vi "RT_init_shared_and_network_variables.vi"(8 "error in (no error)":errorcluster) -> (0 "error out":errorcluster)   [LabVIEW 2020]
uses:
  RT_CPU_load.ctl
  RT_FIFO_Health.ctl
  RT_only_FIFO_Health.ctl
  PC_DIO_Cluster.ctl
panel:
  out "current time":timestamp
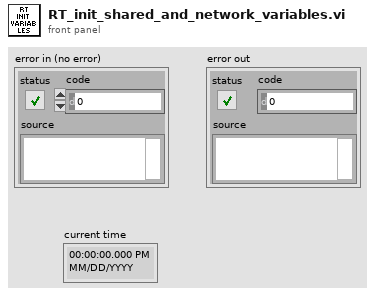
[diagram p1: front panel]
types:
  T1 = typedef "PC_DIO_Cluster.ctl" = cluster{"DIO1":bool, "DIO0":bool, "DIO2":bool, "DIO3":bool}
  T2 = typedef "RT_only_FIFO_Health.ctl" = cluster{"Elements in RT FIFO":i32, "Network Stream Full":bool, "RT FIFO Full":bool, "FPGA AI Underflow":bool, "FPGA FIFO Full":bool, "FPGA Loop Timing Off":bool, "timestamp":timestamp}
  T3 = typedef "RT_FIFO_Health.ctl" = cluster{dbl, dbl, dbl, "TotalPhysMem":dbl, "FreePhysMem":dbl, "TotalVirtMem":dbl, "FreeVirtMem":dbl, "TotalDisk":dbl, "FreeDisk":dbl}
  T4 = typedef "RT_CPU_load.ctl" = cluster{"Total (%)":dbl, "Time Critical (%)":dbl, "Timed Structures (%)":dbl, "High (%)":dbl, "Above Normal (%)":dbl, "Normal (%)":dbl, "Background (%)":dbl, "Idle (%)":dbl, "ISR (%)":dbl, "ISR (%) 2":dbl, "Idle (%) 2":dbl, "Background (%) 2":dbl, "Normal (%) 2":dbl, "Above Normal (%) 2":dbl, "High (%) 2":dbl, "Timed Structures (%) 2":dbl, "Time Critical (%) 2":dbl, "Total (%) 2":dbl}
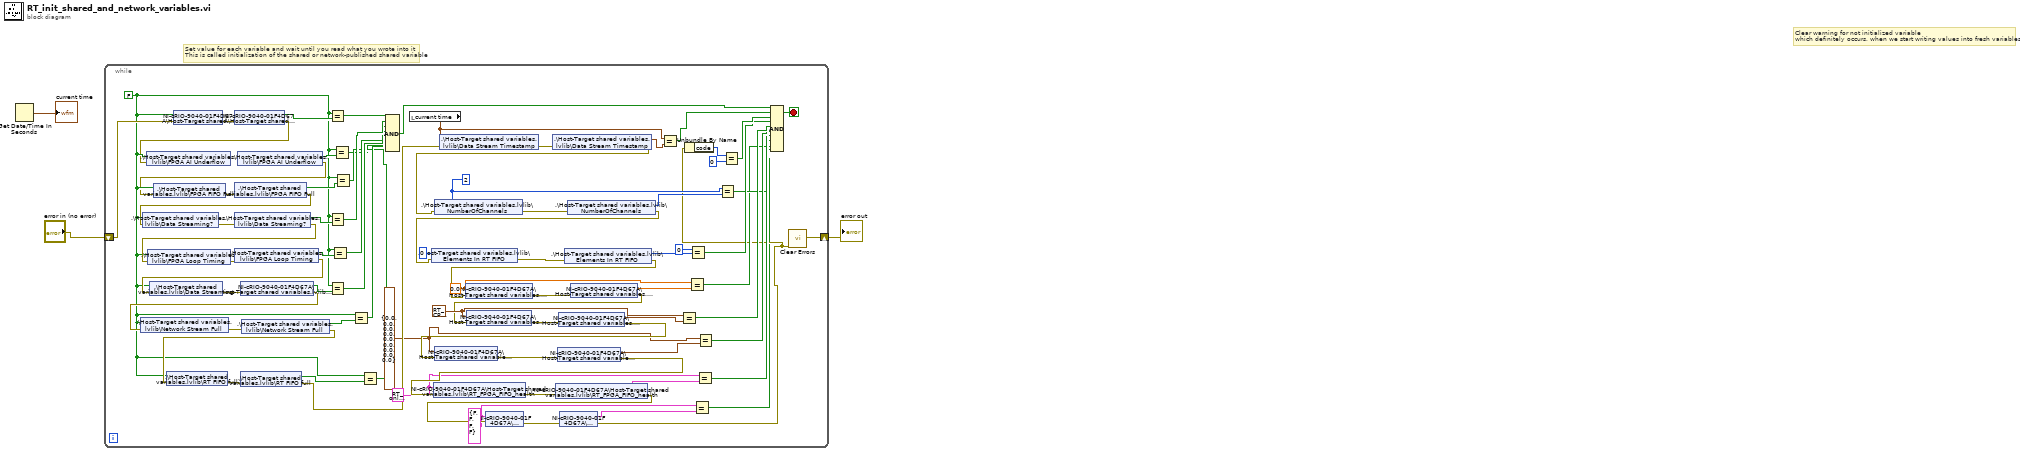
[diagram p0: block diagram]
diagram:
  # "Set value for each variable and wait until you read what you wrote into it\nThis is called initialization of the shared or network-published shared variable"
  # "Clear warning for not initialized variable\nwhich definitely occurs, when we start writing values into fresh variables"
  n1 = Get Date/Time In Seconds() -> (seconds since 1Jan1904=→"current time":timestamp)
  n2 = while {
    shift-right: [w72] -> w2
    shift-left: "error in (no error)" -> [w71]
    stop <- w65 stop-if-true
    w5 = T1 {"DIO1"=FALSE, "DIO0"=FALSE, "DIO2"=FALSE, "DIO3"=FALSE} ("DIO")
    w11 = 0.0 ("Binning Time")
    w31 = u8 2 ("NumberOfChannels")
    w37 = T2 {"Elements in RT FIFO"=0, "Network Stream Full"=FALSE, "RT FIFO Full"=FALSE, "FPGA AI Underflow"=FALSE, "FPGA FIFO Full"=FALSE, "FPGA Loop Timing Off"=FALSE, "timestamp"=timestamp(0 s since 1904-01-01)} ("RT_FIFO_health")
    w43 = T3 {0.0, 0.0, 0.0, "TotalPhysMem"=0.0, "FreePhysMem"=0.0, "TotalVirtMem"=0.0, "FreeVirtMem"=0.0, "TotalDisk"=0.0, "FreeDisk"=0.0} ("RT_FPGA_Memory_and_FIFOs")
    w46 = T4 {"Total (%)"=0.0, "Time Critical (%)"=0.0, "Timed Structures (%)"=0.0, "High (%)"=0.0, "Above Normal (%)"=0.0, "Normal (%)"=0.0, "Background (%)"=0.0, "Idle (%)"=0.0, "ISR (%)"=0.0, "ISR (%) 2"=0.0, "Idle (%) 2"=0.0, "Background (%) 2"=0.0, "Normal (%) 2"=0.0, "Above Normal (%) 2"=0.0, "High (%) 2"=0.0, "Timed Structures (%) 2"=0.0, "Time Critical (%) 2"=0.0, "Total (%) 2"=0.0} ("RT CPU Load")
    w21 = FALSE
    n3 = shared-variable "NI-cRIO-9040-01F4D67A\\Host-Target shared variables.lvlib\\Stop RT"(w21, error in=w71) -> (error out=w82:errorcluster)
    n4 = shared-variable "NI-cRIO-9040-01F4D67A\\Host-Target shared variables.lvlib\\Stop RT"(error in=w82) -> (w81:bool, error out=w19:errorcluster)
    n5 = shared-variable ".\\Host-Target shared variables.lvlib\\FPGA AI Underflow"(w21, error in=w19) -> ()  [unwired: 1 out]
    n6 = shared-variable ".\\Host-Target shared variables.lvlib\\FPGA AI Underflow"() -> (w23:bool, error out=w18:errorcluster)  [unwired: 1 in]
    n7 = shared-variable ".\\Host-Target shared variables.lvlib\\FPGA FIFO Full"(w21, error in=w18) -> (error out=w24:errorcluster)
    n8 = shared-variable ".\\Host-Target shared variables.lvlib\\FPGA FIFO Full"(error in=w24) -> (w22:bool, error out=w20:errorcluster)
    n9 = shared-variable ".\\Host-Target shared variables.lvlib\\Data Streaming?"(w21, error in=w20) -> (error out=w80:errorcluster)
    n10 = shared-variable ".\\Host-Target shared variables.lvlib\\Data Streaming?"(error in=w80) -> (w79:bool, error out=w28:errorcluster)
    n11 = shared-variable ".\\Host-Target shared variables.lvlib\\FPGA Loop Timing"(w21, error in=w28) -> (error out=w29:errorcluster)
    n12 = shared-variable ".\\Host-Target shared variables.lvlib\\FPGA Loop Timing"(error in=w29) -> (w26:bool, error out=w27:errorcluster)
    n13 = shared-variable ".\\Host-Target shared variables.lvlib\\Data Streaming"(w21, error in=w27) -> (error out=w83:errorcluster)
    n14 = shared-variable "NI-cRIO-9040-01F4D67A\\Host-Target shared variables.lvlib\\Data Streaming"(error in=w83) -> (w78:bool, error out=w61:errorcluster)
    n15 = shared-variable ".\\Host-Target shared variables.lvlib\\Network Stream Full"(w21, error in=w61) -> (error out=w63:errorcluster)
    n16 = shared-variable ".\\Host-Target shared variables.lvlib\\Network Stream Full"(error in=w63) -> (w58:bool, error out=w60:errorcluster)
    n17 = shared-variable ".\\Host-Target shared variables.lvlib\\RT FIFO full"(w21, error in=w60) -> (error out=w62:errorcluster)
    n18 = shared-variable ".\\Host-Target shared variables.lvlib\\RT FIFO full"(error in=w62) -> (w57:bool, error out=w59:errorcluster)
    n19 = Equal?(x=w21, y=w81) -> (x = y?=w77:bool)
    n20 = Equal?(x=w21, y=w79) -> (x = y?=w76:bool)
    n21 = Equal?(x=w21, y=w78) -> (x = y?=w75:bool)
    n22 = Equal?(x=w21, y=w26) -> (x = y?=w25:bool)
    n23 = Equal?(x=w21, y=w23) -> (x = y?=w16:bool)
    n24 = Equal?(x=w21, y=w22) -> (x = y?=w17:bool)
    n25 = Equal?(x=w21, y=w58) -> (x = y?=w56:bool)
    n26 = Equal?(x=w21, y=w57) -> (x = y?=w55:bool)
    n27 = Compound Arithmetic op=AND(w77, w76, w75, w56, w55, w25, w16, w17) -> (w68:bool)
    n28 = local read "current time"() -> (w64:timestamp)
    n29 = shared-variable ".\\Host-Target shared variables.lvlib\\Data Stream Timestamp"(w64, error in=w59) -> (error out=w70:errorcluster)
    n30 = shared-variable ".\\Host-Target shared variables.lvlib\\Data Stream Timestamp"(error in=w70) -> (w69:timestamp, error out=w35:errorcluster)
    n31 = shared-variable ".\\Host-Target shared variables.lvlib\\NumberOfChannels"(w31, error in=w35) -> (error out=w34:errorcluster)
    n32 = shared-variable ".\\Host-Target shared variables.lvlib\\NumberOfChannels"(error in=w34) -> (w32:u8, error out=w33:errorcluster)
    n33 = shared-variable ".\\Host-Target shared variables.lvlib\\Elements In RT FIFO"(0 ("Elements In RT FIFO AI"), error in=w33) -> (error out=w54:errorcluster)
    n34 = shared-variable ".\\Host-Target shared variables.lvlib\\Elements In RT FIFO"(error in=w54) -> (w52:i32, error out=w14:errorcluster)
    n35 = shared-variable "NI-cRIO-9040-01F4D67A\\Host-Target shared variables.lvlib\\Binning Time"(w11, error in=w14) -> (error out=w15:errorcluster)
    n36 = shared-variable "NI-cRIO-9040-01F4D67A\\Host-Target shared variables.lvlib\\Binning Time"(error in=w15) -> (w12:dbl, error out=w13:errorcluster)
    n37 = shared-variable "NI-cRIO-9040-01F4D67A\\Host-Target shared variables.lvlib\\RT CPU Load"(w46, error in=w13) -> (error out=w48:errorcluster)
    n38 = shared-variable "NI-cRIO-9040-01F4D67A\\Host-Target shared variables.lvlib\\RT CPU Load"(error in=w48) -> (w45:T4, error out=w47:errorcluster)
    n39 = shared-variable "NI-cRIO-9040-01F4D67A\\Host-Target shared variables.lvlib\\RT_Memory"(w43, error in=w47) -> (error out=w49:errorcluster)
    n40 = shared-variable "NI-cRIO-9040-01F4D67A\\Host-Target shared variables.lvlib\\RT_Memory"(error in=w49) -> (w44:T3, error out=w39:errorcluster)
    n41 = shared-variable "NI-cRIO-9040-01F4D67A\\Host-Target shared variables.lvlib\\RT_FPGA_FIFO_health"(w37, error in=w39) -> (error out=w40:errorcluster)
    n42 = shared-variable "NI-cRIO-9040-01F4D67A\\Host-Target shared variables.lvlib\\RT_FPGA_FIFO_health"(error in=w40) -> (w38:T2, error out=w9:errorcluster)
    n43 = shared-variable "NI-cRIO-9040-01F4D67A\\Host-Target shared variables.lvlib\\DIO"(w5, error in=w9) -> (error out=w8:errorcluster)
    n44 = shared-variable "NI-cRIO-9040-01F4D67A\\Host-Target shared variables.lvlib\\DIO"(error in=w8) -> (w6:T1, error out=w7:errorcluster)
    n45 = Equal?(x=w64, y=w69) -> (x = y?=w67:bool)
    n46 = Equal?(x=w46, y=w45) -> (x = y?=w42:bool)
    n47 = Unbundle By Name(w7) -> ("code"=w74:i32)
    n48 = Equal?(x=w11, y=w12) -> (x = y?=w10:bool)
    n49 = Equal?(x=0, y=w52) -> (x = y?=w50:bool)
    n50 = Equal?(x=w5, y=w6) -> (x = y?=w4:bool)
    n51 = Equal?(x=w37, y=w38) -> (x = y?=w36:bool)
    n52 = Equal?(x=w43, y=w44) -> (x = y?=w41:bool)
    n53 = Equal?(x=w31, y=w32) -> (x = y?=w30:bool)
    n54 = Equal?(x=w74, y=0) -> (x = y?=w66:bool)
    n55 = Compound Arithmetic op=AND(w68, w67, w66, w50, w42, w41, w36, w30, w10, w4) -> (w65:bool)
    n56 = call <vilib>:"Clear Errors.vi"("error in (no error)"=w7) -> ("error out"=w72:errorcluster)  [unwired: 5 in, 1 out]
  }
  "error out" <- w2
